vi "Create.vi"(8 "error in (no error)":errorcluster, 9 "Main Memory Ref":refnum<vi>, 10 "Variable Table Ref":refnum<vi>) -> (0 "error out":errorcluster, 3 "gScript Interpreter out":refnum<class "gScript Interpreter.lvclass">)   [LabVIEW 2017, in "gScript Interpreter.lvclass"]
uses:
  gScript Interpreter.lvclass
  Type Definitions/Main Memory.ctl
  Type Definitions/Memory Cell.ctl
  Type Definitions/Memory Cell Type Enum.ctl
  gScript Interpreter.lvclass/gScript Interpreter.ctl
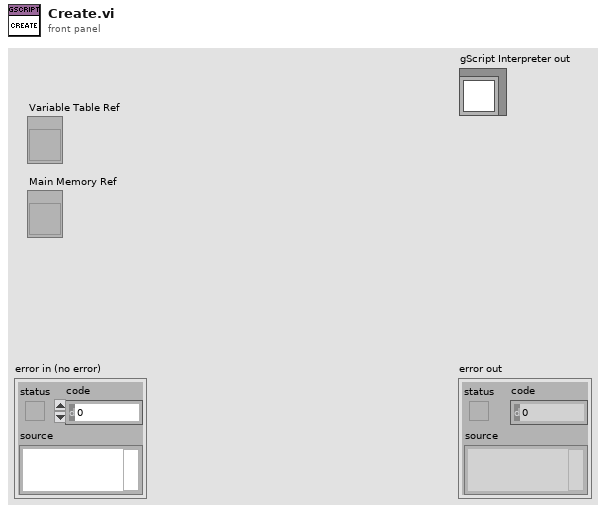
[diagram p1: front panel]
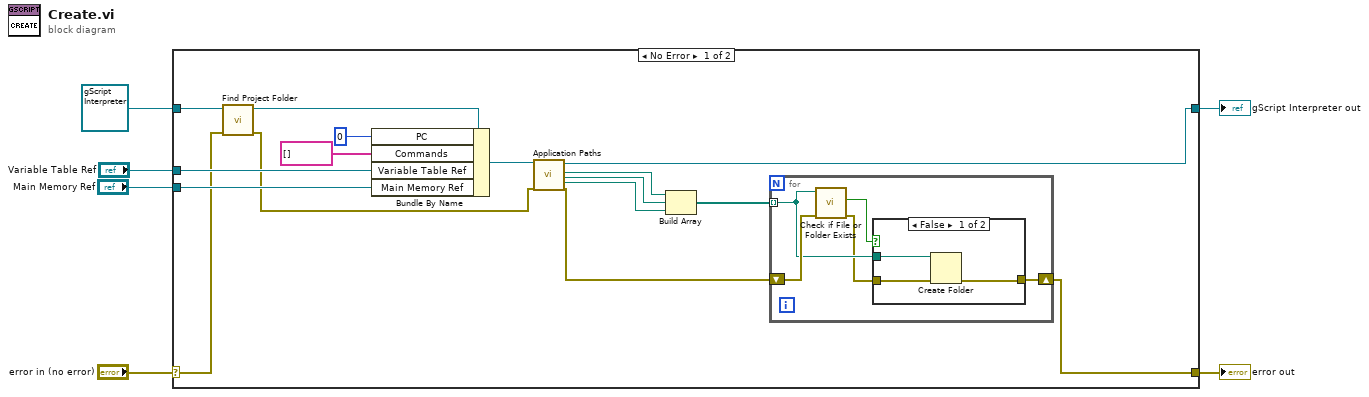
[diagram p0: block diagram]
diagram:
  n1 = case shown="No Error" "error in (no error)" {
    selector: "error in (no error)" -> [w17 w33]
    tunnel: [w7 w33] -> w5
    tunnel: [w8 w32] -> w3
    tunnel: refnum<class "gScript Interpreter.lvclass"> refnum ("gScript Interpreter in") -> [w18 w32]
    tunnel: "Main Memory Ref" -> [w20 _]
    tunnel: "Variable Table Ref" -> [w19 _]
    frame No Error {
      n2 = call "Find Project Folder.vi"("error in (no error)"=w17, "gScript Interpreter in"=w18) -> ("error out"=w14:errorcluster, "gScript Interpreter out"=w16:refnum<class "gScript Interpreter.lvclass">)  [unwired: 8 in]
      n3 = Bundle By Name(cluster=w16, "PC"=0, "Commands"=string[] [], "Variable Table Ref"=w19, "Main Memory Ref"=w20) -> (w15:refnum<class "gScript Interpreter.lvclass">)
      n4 = call "Application Paths.vi"("gScript Interpreter in"=w15, "error in (no error)"=w14) -> ("gScript Interpreter out"=w8:refnum<class "gScript Interpreter.lvclass">, "Config Path"=w13:path, "Scripts Path"=w12:path, "Logs Path"=w11:path, "error out"=w9:errorcluster)  [unwired: 12 in, 1 out]
      n5 = Build Array(w13, w12, w11) -> (w10:path[])
      n6 = for {
        tunnel: w10 -> [w25] mode=indexing
        shift-right: [w23] -> w7
        shift-left: w9 -> [w27]
        n7 = call <vilib>:"Check if File or Folder Exists.vi"("error in (no error)"=w27, "path"=w25) -> ("error out"=w24:errorcluster, "file or folder exists?"=w26:bool)  [unwired: 7 in, 1 out]
        n8 = case shown="False" w26 {
          tunnel: w25 -> [w30 _]
          tunnel: w24 -> [w29 w31]
          tunnel: [w28 w31] -> w23
          frame False {
            n9 = Create Folder(path (use dialog)=w30, error in=w29) -> (error out=w28:errorcluster)  [unwired: 1 in, 2 out]
          }
          frame True {
          }
        }
      }
    }
    frame Error {
    }
  }
  "error out" <- w5
  "gScript Interpreter out" <- w3
